vi "Main.vi"(11 "Module Admin":refnum<class "Delacor_lib_QMH_Module Admin.lvclass">) -> ()   [LabVIEW 2020, in "Acquisition.lvlib"]
doc: "This template is based off of the Queued Message Handler design pattern and the Queued Message Handler project template that ships with LabVIEW.\n\nThe main difference is that the queue is private to this module and communication between modules is performed via Broadcast and Request events.\n\nRequest events are wrapped in public API methods and are handled in the Event Handling Loop (EHL) of this VI. Any module can register for Broadcast events sent by this module. The EHL generates messages based on user interface actions.\n\nThe Message Handling Loop (MHL) processes messages generated by the EHL, or by other messages. The messages are string values, so new messages can be added easily to the Message Cases case structure in the MHL. Each message cluster can also provide an optional value for Message Data, which is a variant that can be converted to whatever message-specific data is required.\n_____\nBased on Delacor QMH Project Template 6.0.0.89."
uses:
  Acquisition.lvlib
  <vilib>/Delacor/Delacor QMH/Libraries/Module Admin_class/Delacor_lib_QMH_Module Admin.lvclass
  Shared/AnalogAcquisitionParameters__typedef.ctl
  Shared/DigitalAcquisitionParameters__typedef.ctl
  Module Data--cluster.ctl
  Stop Argument--cluster.ctl
  <vilib>/Delacor/Delacor QMH/Libraries/Message Queue_class/Delacor_lib_QMH_Message Queue.lvclass/Delacor_lib_QMH_Message Queue.ctl
  <vilib>/Delacor/Delacor QMH/Libraries/Module Admin_class/Delacor_lib_QMH_Module Admin.lvclass/Delacor_lib_QMH_Module Admin.ctl
  Start Acquisition Argument--cluster.ctl
  Configure Analog Task Acquisition Argument--cluster.ctl
  Configure Digital Taks Acquisition Argument--cluster.ctl
  Start Analog Acquisition Helper Loop Argument--cluster.ctl
  Start Digital Acquisition Helper Loop Argument--cluster.ctl
  Stop Analog Acquisition Helper Loop Argument--cluster.ctl
  Stop Digital Acquisition Helper Loop Argument--cluster.ctl
  <vilib>/DAQmx/read.llb/DAQmx Read (Digital 1D U32 NChan 1Samp).vi
  <vilib>/DAQmx/read.llb/DAQmx Read (Digital 1D Bool NChan 1Samp 1Line).vi
  <vilib>/DAQmx/read.llb/DAQmx Read (Analog 1D Wfm NChan NSamp).vi
  <vilib>/Delacor/Delacor QMH/Libraries/Message Queue_class/Delacor_lib_QMH_Enqueue Message (Single).vi
  <vilib>/Delacor/Delacor QMH/Libraries/Module Admin_class/Delacor_lib_QMH_Get External Launch.vi
  <vilib>/DAQmx/miscellaneous.llb/DAQmx Fill In Error Info.vi
  <vilib>/Utility/error.llb/Error Cluster From Error Code.vi
  <vilib>/ErrorRing/Error Ring.xnode
  <vilib>/Delacor/Delacor QMH/Libraries/Message Queue_class/Delacor_lib_QMH_Message Queue.lvclass
  Shared/Configuration for Acquisitions.lvlib
panel:
  in  "Analog - Digital":bool
  in  "Digital Acquisition Parameters":T1 {"Execution Task Frequency" scale=1.0..100.0}
  in  "Analog Acquisition Parameters":T2={"sampling frequency Analog"=1000, "number of samples Analog"=1000, "Channels Analog"=[]} {"number of samples Analog" scale=0.0..2000.0; "sampling frequency Analog" scale=0.0..2000.0}
  in  "Total Acquisition Time":i32
  in  "DAQ Device Name":tag
  out "error out":errorcluster
  in  "Start Acquisition":bool
  out "Array Datos Digitales":bool[](array[boolean])
  out "Grafica Datos Analógicos":waveform(dbl)[](graph)
  out "Status":string
  # "#LaterOn\nThis parameters are not taken from the Acquisition module, but\nreceived by it. The information comes from an external request\n(tester) or from a broadcast (Settings module)"
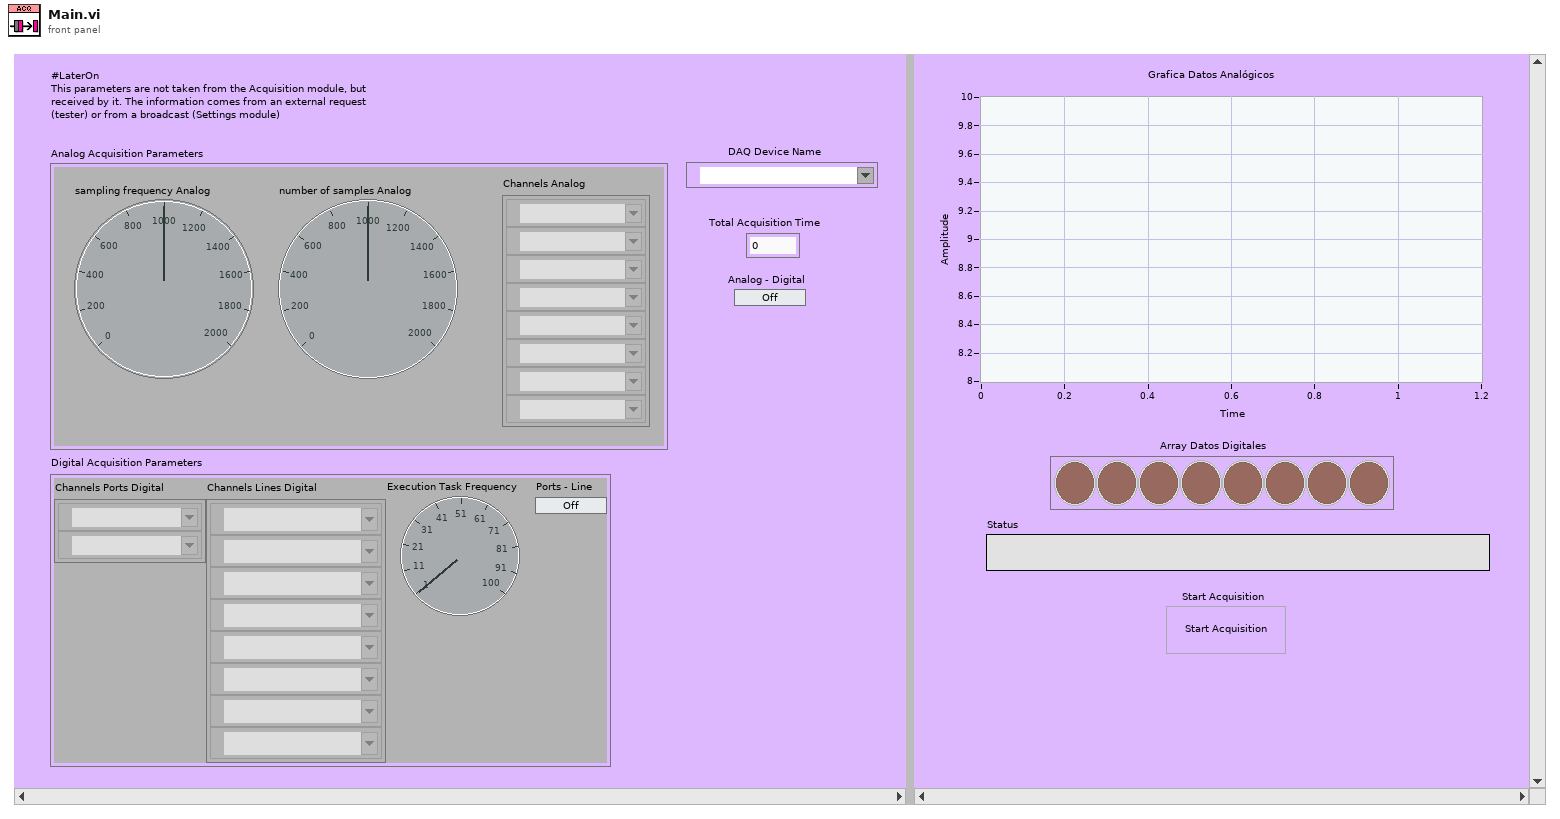
[diagram p1: front panel]
types:
  T1 = typedef "Configuration for Acquisitions.lvlib/DigitalAcquisitionParameters__typedef.ctl" = cluster{"Channels Ports Digital":tag[], "Channels Lines Digital":tag[], "Execution Task Frequency\n":u32, "Ports - Line":bool}
  T2 = typedef "Configuration for Acquisitions.lvlib/AnalogAcquisitionParameters__typedef.ctl" = cluster{"sampling frequency Analog":u32, "number of samples Analog":u32, "Channels Analog":tag[]}
  T3 = typedef "Acquisition.lvlib/Request Events--cluster.ctl" = cluster{"Stop Module":refnum<user-event>, "Show Panel":refnum<user-event>, "Hide Panel":refnum<user-event>, "Get Module Execution Status":refnum<user-event>, "Show Diagram":refnum<user-event>, "Start Acquisition":refnum<user-event>, "Configure Analog Task Acquisition":refnum<user-event>, "Configure Digital Taks Acquisition":refnum<user-event>, "Start Analog Acquisition Helper Loop":refnum<user-event>, "Start Digital Acquisition Helper Loop":refnum<user-event>, "Stop Analog Acquisition Helper Loop":refnum<user-event>, "Stop Digital Acquisition Helper Loop":refnum<user-event>}
  T4 = enum32{"invalid lock state", "Not Locked", "Locked (No Password)", "Password-protected"}
  T5 = typedef "Acquisition.lvlib/Stop Argument--cluster.ctl" = cluster{"Origin":string, "Exit via Stop Module Req?":bool, "Wait for Module to stop?":bool}
  T6 = typedef "Acquisition.lvlib/Start Acquisition Argument--cluster.ctl" = cluster{"Start Acquisition":bool, "Analog - Digital":bool}
  T7 = typedef "Acquisition.lvlib/Configure Analog Task Acquisition Argument--cluster.ctl" = cluster{"DAQ Device Name":tag, "Total Acquisition Time":i32, "Analog Acquisition Parameters":T2}
  T8 = typedef "Acquisition.lvlib/Configure Digital Taks Acquisition Argument--cluster.ctl" = cluster{"DAQ Device Name":tag, "Total Acquisition Time":i32, "Digital Acquisition Parameters":T1}
  T9 = typedef "Acquisition.lvlib/Start Analog Acquisition Helper Loop Argument--cluster.ctl" = cluster{"Analog Acq. Timeout":i32}
  T10 = typedef "Acquisition.lvlib/Start Digital Acquisition Helper Loop Argument--cluster.ctl" = cluster{"Digital Acq. Timeout":i32}
  T11 = typedef "Acquisition.lvlib/Stop Analog Acquisition Helper Loop Argument--cluster.ctl" = cluster{"Boolean":bool}
  T12 = typedef "Acquisition.lvlib/Stop Digital Acquisition Helper Loop Argument--cluster.ctl" = cluster{"Boolean":bool}
  T13 = enum32{"Invalid", "Standard", "Closed", "Hidden", "Minimized", "Maximized"}
  T14 = typedef "Acquisition.lvlib/Module Data--cluster.ctl" = cluster{"Status":string, "DAQ Device Name":tag, "Total Acquisition Time":u32, "Analog Acquisition Parameters":T2, "Digital Acquisition Parameters":T1, "Acquisition Type":bool}
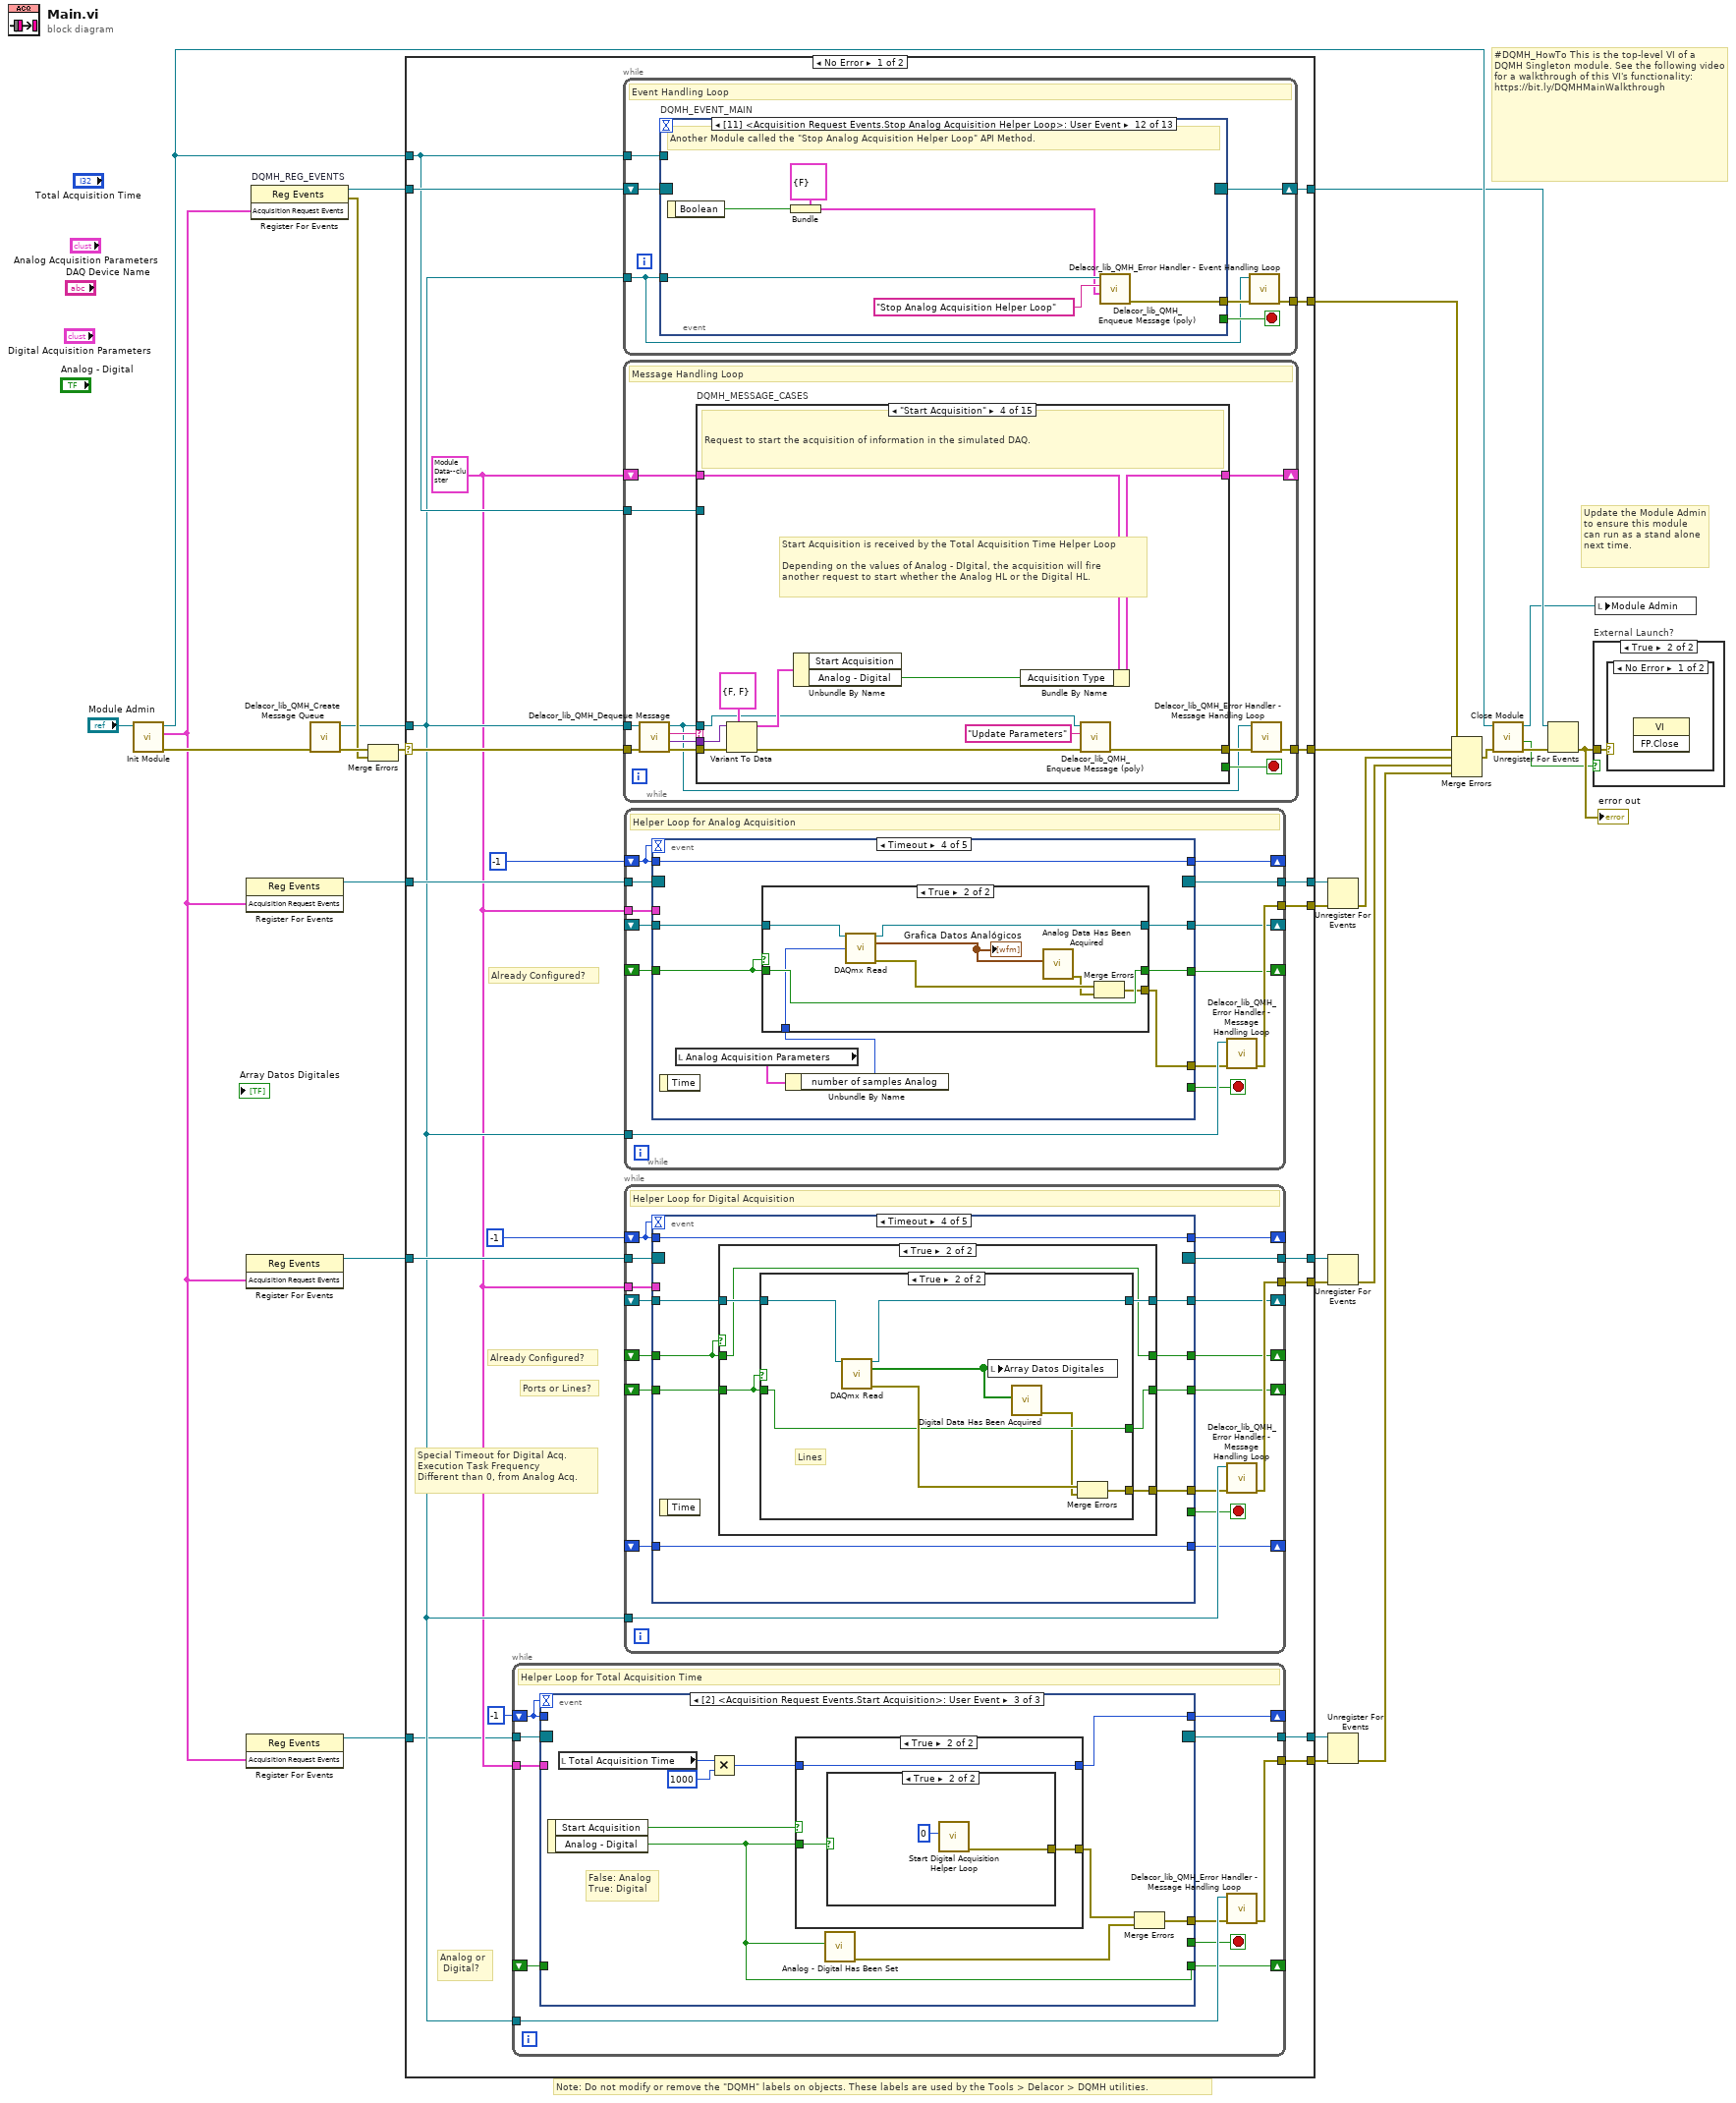
[diagram p0: block diagram]
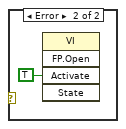
[diagram p3: hidden frame]
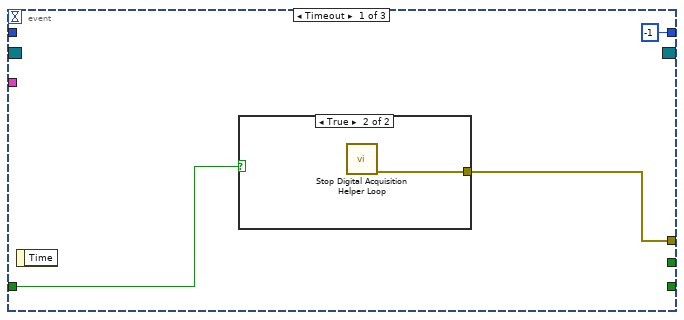
[diagram p4: hidden frame]
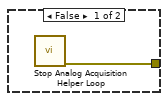
[diagram p5: hidden frame]
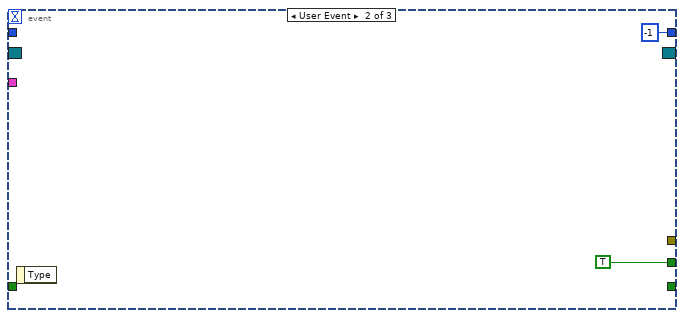
[diagram p6: hidden frame]
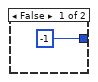
[diagram p7: hidden frame]
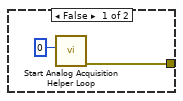
[diagram p8: hidden frame]
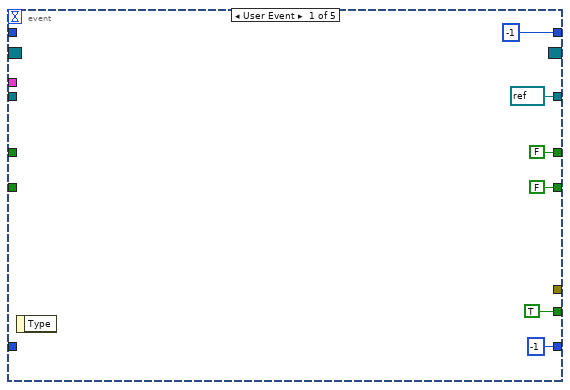
[diagram p9: hidden frame]
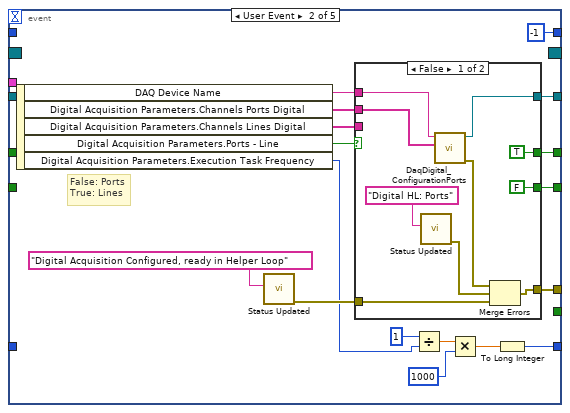
[diagram p10: hidden frame]
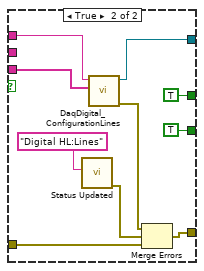
[diagram p11: hidden frame]
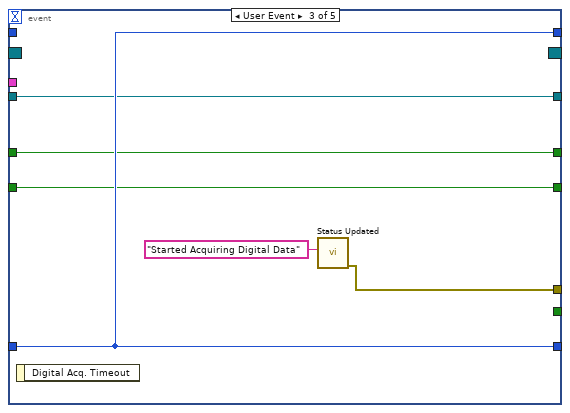
[diagram p12: hidden frame]
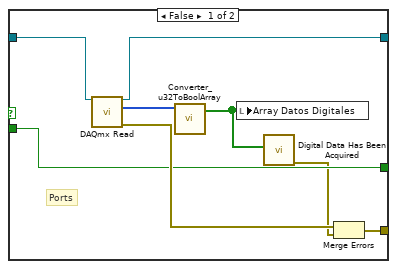
[diagram p14: hidden frame]
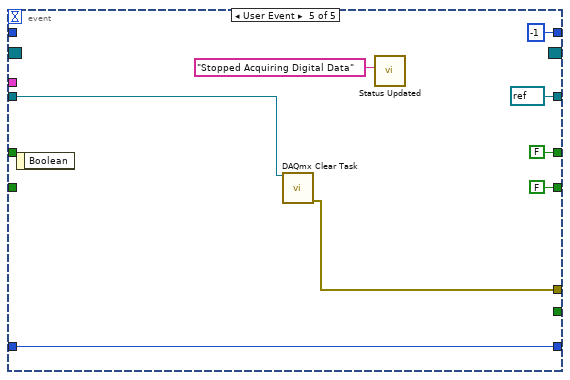
[diagram p15: hidden frame]
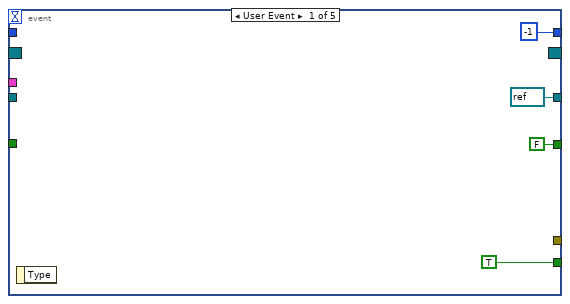
[diagram p16: hidden frame]
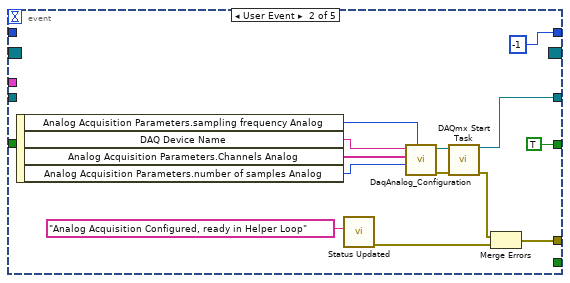
[diagram p17: hidden frame]
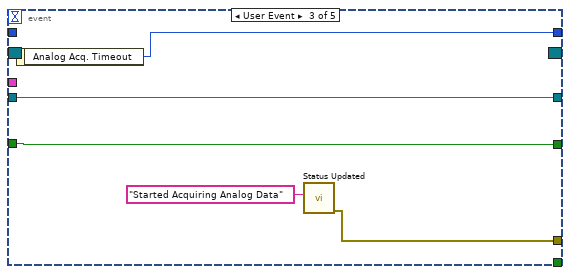
[diagram p18: hidden frame]
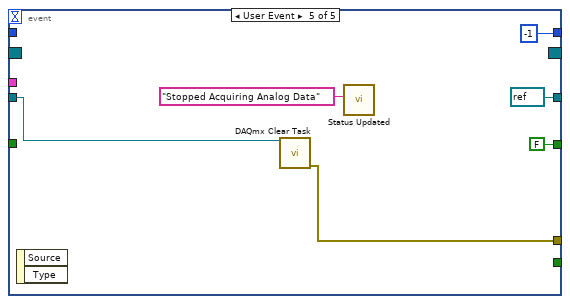
[diagram p20: hidden frame]
diagram:
  # "#DQMH_HowTo This is the top-level VI of a DQMH Singleton module. See the following video for a walkthrough of this VI's functionality: https://bit.ly/DQMHMainWalkthrough"
  # "Note: Do not modify or remove the \"DQMH\" labels on objects. These labels are used by the Tools > Delacor > DQMH utilities."
  # "Update the Module Admin to ensure this module can run as a stand alone next time."
  n1 = call "Init Module.vi"("Singleton Module Admin in"="Module Admin") -> ("error out"=w28:errorcluster, "Acquisition Request Events"=w1:T3, "Singleton Module Admin out"=w20:refnum<class "Delacor_lib_QMH_Module Admin.lvclass">)  [unwired: 8 in]
  n2 = register-events(w1) -> (reference out=w13:refnum<event-registration>)  [unwired: 2 in, 1 out]
  n3 = register-events(w1) -> (reference out=w9:refnum<event-registration>)  [unwired: 2 in, 1 out]
  n4 = register-events(w1) -> (reference out=w2:refnum<event-registration>)  [unwired: 2 in, 1 out]
  n5 = register-events "DQMH_REG_EVENTS"(w1) -> (reference out=w18:refnum<event-registration>, error out=w21:errorcluster)  [unwired: 2 in]
  n6 = call <vilib>:"Delacor_lib_QMH_Create Message Queue.vi"("error in"=w28) -> ("error out"=w23:errorcluster, "Message Queue"=w17:refnum<class "Delacor_lib_QMH_Message Queue.lvclass">)  [unwired: 9 in]
  n7 = Merge Errors(w23, w21) -> (w22:errorcluster)
  n8 = case shown="No Error" w22 {
    selector: w22 -> [w47 w507]
    tunnel: [w49 w506] -> w29
    tunnel: [w46 w512] -> w19
    tunnel: w18 -> [w45 w512]
    tunnel: w17 -> [w36 w505]
    tunnel: [w48 _] -> w26
    tunnel: w20 -> [w41 w508]
    tunnel: w13 -> [w44 w504]
    tunnel: [w43 w504] -> w12
    tunnel: [w42 _] -> w11
    tunnel: w9 -> [w40 w503]
    tunnel: [w39 w503] -> w8
    tunnel: [w38 _] -> w7
    tunnel: [w34 w502] -> w5
    tunnel: [w33 _] -> w4
    tunnel: w2 -> [w32 w502]
    frame No Error {
      w35 = T14 {"Status"="", "DAQ Device Name"="", "Total Acquisition Time"=0, "Analog Acquisition Parameters"={"sampling frequency Analog"=1000, "number of samples Analog"=1000, "Channels Analog"=[]}, "Digital Acquisition Parameters"={"Channels Ports Digital"=[], "Channels Lines Digital"=[], "Execution Task Frequency\n"=0, "Ports - Line"=FALSE}, "Acquisition Type"=FALSE} ("Data Cluster")
      # "Analog or\n Digital?"
      # "Ports or Lines?"
      # "Special Timeout for Digital Acq.\nExecution Task Frequency\nDifferent than 0, from Analog Acq."
      # "Already Configured?"
      # "Already Configured?"
      n9 = while {
        tunnel: w32 -> [w60]
        shift-right: [w58] -> _
        shift-left: -1 -> [w59]
        tunnel: w35 -> [w57]
        tunnel: [w56] -> w34
        tunnel: [w55] -> w33
        tunnel: w36 -> [w54]
        shift-right: [w51] -> _
        shift-left: _ -> [w50]
        stop <- w52 stop-if-true
        # "Helper Loop for Total Acquisition Time"
        n10 = event shown="[2] <Acquisition Request Events.Start Acquisition>: User Event" {
          selector: w60 -> [_ _ _]
          dyn-events: [_ _ _] -> w56
          timeout: w59 -> [_ _ _]
          tunnel: w59 -> [_ _ _]
          tunnel: [-1 -1 w73] -> w58
          tunnel: w57 -> [_ _ _]
          tunnel: [w62 _ w69] -> w53
          tunnel: [_ TRUE _] -> w52
          tunnel: [_ _ w70] -> w51
          tunnel: w50 -> [w63 _ _]
          event Timeout {
            n11 = event-data() -> ()  [unwired: 1 in, 1 out]
            n12 = case shown="True" w63 {
              tunnel: [w64 w65] -> w62
              frame False {
                n13 = call "Stop Analog Acquisition Helper Loop.vi"() -> ("error out"=w64:errorcluster)  [unwired: 11 in]
              }
              frame True {
                n14 = call "Stop Digital Acquisition Helper Loop.vi"() -> ("error out"=w65:errorcluster)  [unwired: 11 in]
              }
            }
          }
          event User Event {
            n15 = event-data() -> ()  [unwired: 1 in, 1 out]
          }
          event User Event {
            # "False: Analog\nTrue: Digital"
            n16 = event-data() -> ("Start Acquisition"=w76:bool, "Analog - Digital"=w70:bool)  [unwired: 1 in]
            n17 = local read "Total Acquisition Time"() -> (w74:i32)
            n18 = Multiply(x=w74, y=1000) -> (x*y=w72:i32)
            n19 = case shown="True" w76 {
              tunnel: w70 -> [_ w80]
              tunnel: [_ w79] -> w75
              tunnel: w72 -> [_ w78]
              tunnel: [-1 w78] -> w73
              frame False {
              }
              frame True {
                n20 = case shown="True" w80 {
                  tunnel: [w82 w84] -> w79
                  frame False {
                    n21 = call "Start Analog Acquisition Helper Loop.vi"("Analog Acq. Timeout"=0) -> ("error out"=w82:errorcluster)  [unwired: 10 in]
                  }
                  frame True {
                    n22 = call "Start Digital Acquisition Helper Loop.vi"("Digital Acq. Timeout"=0) -> ("error out"=w84:errorcluster)  [unwired: 10 in]
                  }
                }
              }
            }
            n23 = call "Analog - Digital Has Been Set.vi"("Analog - Digital"=w70) -> ("error out"=w68:errorcluster)  [unwired: 10 in]
            n24 = Merge Errors(w75, w68) -> (w69:errorcluster)
          }
        }
        n25 = call-dynamic "Delacor_lib_QMH_Error Handler - Message Handling Loop.vi"("error in"=w53, "Message Queue in"=w54) -> ("dup error in"=w55:errorcluster)  [unwired: 8 in, 1 out]
      }
      n26 = while {
        tunnel: w36 -> [w251]
        shift-right: [w254] -> w46
        shift-left: w45 -> [w255]
        tunnel: [w256] -> w48
        tunnel: w41 -> [w252]
        stop <- w253 stop-if-true
        # "Event Handling Loop"
        n27 = event "DQMH_EVENT_MAIN" shown="[11] <Acquisition Request Events.Stop Analog Acquisition Helper Loop>: User Event" {
          selector: w255 -> [_ _ _ _ _ _ _ _ _ _ _ _ _]
          dyn-events: [_ _ _ _ _ _ _ _ _ _ _ _ _] -> w254
          timeout: _ -> [_ _ _ _ _ _ _ _ _ _ _ _ _]
          tunnel: [_ _ _ _ TRUE ("Discard?") _ _ _ _ _ _ _ _] -> w253
          tunnel: w251 -> [_ _ _ _ w280 w287 w301 w309 w317 w323 w329 w335 w341]
          tunnel: [_ _ w263 _ w283 w289 w296 w302 w310 w318 w324 w330 w336] -> w257
          tunnel: w252 -> [_ _ _ _ _ w286 _ _ _ _ _ _ _]
          event User Event {
            # "Show the panel of this VI, and send a status updated message to let listeners know."
            # "Another Module called the \"Show Panel\" API Method."
            n28 = event-data() -> ()  [unwired: 1 in, 1 out]
            n29 = control-ref of="This VI"() -> (w259:refnum<vi>)
            n30 = call "Open VI Panel.vi"("VI"=w259) -> ()  [unwired: 10 in, 1 out]
            n31 = call "Status Updated.vi"("Status"="Panel shown." ("format string")) -> ()  [unwired: 10 in, 1 out]
          }
          event User Event {
            # "Hide the panel of this VI, and send a status updated message to let listeners know."
            # "Another Module called the \"Hide Panel\" API Method."
            n32 = event-data() -> ()  [unwired: 1 in, 1 out]
            n33 = control-ref of="This VI"() -> (w261:refnum<vi>)
            n34 = call "Hide VI Panel.vi"("VI"=w261) -> ()  [unwired: 10 in, 1 out]
            n35 = call "Status Updated.vi"("Status"="Panel hidden." ("format string")) -> ()  [unwired: 10 in, 1 out]
          }
          event User Event {
            # "Another Module called the \"Get Module Execution Status\" API Method."
            n36 = event-data() -> ()  [unwired: 1 in, 1 out]
            n37 = call "Update Module Execution Status.vi"("Running?"=TRUE) -> ("error out"=w263:errorcluster)  [unwired: 10 in]
          }
          event User Event {
            # "Another Module called the \"Show Diagram\" API Method. This event is used for debugging."
            n38 = event-data() -> ()  [unwired: 1 in, 1 out]
            n39 = disable-structure shown="RUN_TIME_ENGINE==False" {
              frame condition #0 (active) {
                # "functionality not available in exe"
                n40 = invoke class="VI" method="Lock State.Get"() -> (error out=w269:errorcluster, "Get Lock State"=w268:T4, "pwd in cache"=w265:bool)  [unwired: 4 in, 1 out]
                n41 = Equal?(x=T4."Password-protected", y=w268) -> (x = y?=w266:bool)
                n42 = Compound Arithmetic op=AND(w266, invert w265) -> (w264:bool)
                n43 = case shown="False" w264 {
                  tunnel: w269 -> [w272 _]
                  frame False {
                    n44 = property class="VI"(error in=w272, "BDWin.Open"=TRUE ("Block Diagram Window:Open")) -> ()  [unwired: 1 in, 2 out]
                    n45 = call "Status Updated.vi"("Status"="Block Diagram shown." ("format string")) -> ()  [unwired: 10 in, 1 out]
                  }
                  frame True {
                    # "Password-protected VI, and the password is not in the cache. Do not show the diagram."
                  }
                }
              }
              frame condition #1 {
              }
            }
          }
          event User Event {
            # "The Stop Module Event can get fired from the Exit message in the MHL. The queue gets destroyed in that case. If the queue no longer exists, the Enqueue Exit as a priority message will return error 1. It is safe to ignore, because the module is already exiting."
            # "Another Module called the \"Stop Module\" API Method  or the Message Handling Loop below."
            n46 = event-data() -> ("Origin"=w279:string, "Exit via Stop Module Req?"=w275:bool, "Wait for Module to stop?"=w274:bool)  [unwired: 1 in]
            n47 = local write "Status"(w279) -> ()
            n48 = Bundle By Name(cluster=T5 {"Origin"="", "Exit via Stop Module Req?"=FALSE, "Wait for Module to stop?"=FALSE} ("Stop Argument"), "Exit via Stop Module Req?"=w275, "Wait for Module to stop?"=w274) -> (w273:T5)
            n49 = call-poly <vilib>:"Delacor_lib_QMH_Enqueue Message (poly).vi"("Priority Message? (F)"=TRUE, "Message Data"=w273, "Message"="Exit", "Message Queue in"=w280) -> ("error out"=w284:errorcluster)  [unwired: 6 in, 1 out]
            n50 = call <vilib>:"Clear Errors.vi"("error in (no error)"=w284, "specific error code to clear (0: all)"=1) -> ("error out"=w283:errorcluster)  [unwired: 4 in, 1 out]
          }
          event Panel Close? {
            w288 = TRUE  # Discard the event, the MHL is responsible for closing and stopping this VI.
            # "Hide the panel or send the 'Exit' message if the user clicks the 'X' on the module main VI panel."
            n51 = event-data() -> ()  [unwired: 1 in, 1 out]
            n52 = property class="Module Admin"(reference=w286) -> ("Accessors:External Launch"=w285:bool)  [unwired: 1 in, 2 out]
            n53 = case shown="False" w285 {
              tunnel: w287 -> [_ w293]
              tunnel: [_ w294] -> w289
              frame True {
                # "If externally launched, clicking the 'X' hides the panel, but doesn't close it."
                n54 = control-ref of="This VI"() -> (w290:refnum<vi>)
                n55 = call "Hide VI Panel.vi"("VI"=w290) -> ()  [unwired: 10 in, 1 out]
              }
              frame False {
                # "If run as a stand-alone VI, clicking the panel 'X' stops the VI."
                n56 = call-poly <vilib>:"Delacor_lib_QMH_Enqueue Message (poly).vi"("Priority Message? (F)"=TRUE, "Message"="Exit", "Message Queue in"=w293) -> ("error out"=w294:errorcluster)  [unwired: 7 in, 1 out]
              }
            }
            n57 = event-data("Discard?"=w288) -> ()  [unwired: 1 in, 1 out]
          }
          event User Event {
            # "Another Module called the \"Start Acquisition\" API Method."
            n58 = event-data() -> ("Start Acquisition"=w297:bool, "Analog - Digital"=w295:bool)  [unwired: 1 in]
            n59 = Bundle(cluster=T6 {"Start Acquisition"=FALSE, "Analog - Digital"=FALSE} ("Start Acquisition Argument"), "Start Acquisition"=w297, "Analog - Digital"=w295) -> (w298:T6)
            n60 = call-poly <vilib>:"Delacor_lib_QMH_Enqueue Message (poly).vi"("Message Data"=w298, "Message"="Start Acquisition", "Message Queue in"=w301) -> ("error out"=w296:errorcluster)  [unwired: 7 in, 1 out]
          }
          event User Event {
            # "Another Module called the \"Configure Analog Task Acquisition\" API Method."
            n61 = event-data() -> ("DAQ Device Name"=w305:tag, "Total Acquisition Time"=w304:i32, "Analog Acquisition Parameters"=w303:T2)  [unwired: 1 in]
            n62 = Bundle(cluster=T7 {"DAQ Device Name"="", "Total Acquisition Time"=0, "Analog Acquisition Parameters"={"sampling frequency Analog"=1000, "number of samples Analog"=1000, "Channels Analog"=[]}} ("Configure Analog Task Acquisition Argument"), "DAQ Device Name"=w305, "Total Acquisition Time"=w304, "Analog Acquisition Parameters"=w303) -> (w306:T7)
            n63 = call-poly <vilib>:"Delacor_lib_QMH_Enqueue Message (poly).vi"("Message Data"=w306, "Message"="Configure Analog Task Acquisition", "Message Queue in"=w309) -> ("error out"=w302:errorcluster)  [unwired: 7 in, 1 out]
          }
          event User Event {
            # "Another Module called the \"Configure Digital Taks Acquisition\" API Method."
            n64 = event-data() -> ("DAQ Device Name"=w313:tag, "Total Acquisition Time"=w312:i32, "Digital Acquisition Parameters"=w311:T1)  [unwired: 1 in]
            n65 = Bundle(cluster=T8 {"DAQ Device Name"="", "Total Acquisition Time"=0, "Digital Acquisition Parameters"={"Channels Ports Digital"=[], "Channels Lines Digital"=[], "Execution Task Frequency\n"=0, "Ports - Line"=FALSE}} ("Configure Digital Taks Acquisition Argument"), "DAQ Device Name"=w313, "Total Acquisition Time"=w312, "Digital Acquisition Parameters"=w311) -> (w314:T8)
            n66 = call-poly <vilib>:"Delacor_lib_QMH_Enqueue Message (poly).vi"("Message Data"=w314, "Message"="Configure Digital Taks Acquisition", "Message Queue in"=w317) -> ("error out"=w310:errorcluster)  [unwired: 7 in, 1 out]
          }
          event User Event {
            # "Another Module called the \"Start Analog Acquisition Helper Loop\" API Method."
            n67 = event-data() -> ("Analog Acq. Timeout"=w319:i32)  [unwired: 1 in]
            n68 = Bundle(cluster=T9 {"Analog Acq. Timeout"=0} ("Start Analog Acquisition Helper Loop Argument"), "Analog Acq. Timeout"=w319) -> (w320:T9)
            n69 = call-poly <vilib>:"Delacor_lib_QMH_Enqueue Message (poly).vi"("Message Data"=w320, "Message"="Start Analog Acquisition Helper Loop", "Message Queue in"=w323) -> ("error out"=w318:errorcluster)  [unwired: 7 in, 1 out]
          }
          event User Event {
            # "Another Module called the \"Start Digital Acquisition Helper Loop\" API Method."
            n70 = event-data() -> ("Digital Acq. Timeout"=w325:i32)  [unwired: 1 in]
            n71 = Bundle(cluster=T10 {"Digital Acq. Timeout"=0} ("Start Digital Acquisition Helper Loop Argument"), "Digital Acq. Timeout"=w325) -> (w326:T10)
            n72 = call-poly <vilib>:"Delacor_lib_QMH_Enqueue Message (poly).vi"("Message Data"=w326, "Message"="Start Digital Acquisition Helper Loop", "Message Queue in"=w329) -> ("error out"=w324:errorcluster)  [unwired: 7 in, 1 out]
          }
          event User Event {
            # "Another Module called the \"Stop Analog Acquisition Helper Loop\" API Method."
            n73 = event-data() -> ("Boolean"=w331:bool)  [unwired: 1 in]
            n74 = Bundle(cluster=T11 {"Boolean"=FALSE} ("Stop Analog Acquisition Helper Loop Argument"), "Boolean"=w331) -> (w332:T11)
            n75 = call-poly <vilib>:"Delacor_lib_QMH_Enqueue Message (poly).vi"("Message Data"=w332, "Message"="Stop Analog Acquisition Helper Loop", "Message Queue in"=w335) -> ("error out"=w330:errorcluster)  [unwired: 7 in, 1 out]
          }
          event User Event {
            # "Another Module called the \"Stop Digital Acquisition Helper Loop\" API Method."
            n76 = event-data() -> ("Boolean"=w337:bool)  [unwired: 1 in]
            n77 = Bundle(cluster=T12 {"Boolean"=FALSE} ("Stop Digital Acquisition Helper Loop Argument"), "Boolean"=w337) -> (w338:T12)
            n78 = call-poly <vilib>:"Delacor_lib_QMH_Enqueue Message (poly).vi"("Message Data"=w338, "Message"="Stop Digital Acquisition Helper Loop", "Message Queue in"=w341) -> ("error out"=w336:errorcluster)  [unwired: 7 in, 1 out]
          }
        }
        n79 = call-dynamic "Delacor_lib_QMH_Error Handler - Event Handling Loop.vi"("error in"=w257, "Message Queue in"=w251) -> ("dup error in"=w256:errorcluster)  [unwired: 8 in, 1 out]
      }
      n80 = while {
        tunnel: w36 -> [w344]
        shift-right: [w348] -> _
        shift-left: w35 -> [w349]
        tunnel: w47 -> [w352]
        tunnel: [w350] -> w49
        tunnel: w41 -> [w342]
        stop <- w347 stop-if-true
        # "Message Handling Loop"
        n81 = call-dynamic "Delacor_lib_QMH_Dequeue Message.vi"("error in"=w352, "Message Queue in"=w344) -> ("error out"=w351:errorcluster, "Message Data"=w345:variant, "Message"=w346:string, "Message Queue out"=w343:refnum<class "Delacor_lib_QMH_Message Queue.lvclass">)  [unwired: 6 in]
        n82 = case "DQMH_MESSAGE_CASES" shown="\"Start Acquisition\"" w346 {
          selector: w346 -> [_ _ _ _ _ _ _ _ _ _ _ _ _ _ w489]
          tunnel: w343 -> [_ _ _ w385 w399 w416 _ _ _ _ _ _ w459 w481 _]
          tunnel: w351 -> [w370 w376 w384 w395 w411 w427 w433 w439 w445 w451 w454 w456 w466 w487 w491]
          tunnel: [w368 w376 w384 w387 w397 w413 w431 w437 w443 w449 w453 w456 w462 w484 w492] -> w353
          tunnel: w349 -> [w359 w375 w383 w391 w407 w423 w432 w438 w444 w450 w452 w455 w461 w480 w490]
          tunnel: [w358 w375 w383 w389 w406 w419 w432 w438 w444 w450 w452 w455 w461 w480 w490] -> w348
          tunnel: [_ _ _ _ _ _ _ _ _ _ _ _ _ w479 _] -> w347
          tunnel: w345 -> [_ _ _ w394 w410 w426 w430 w436 w442 w448 _ _ w460 w478 _]
          tunnel: w342 -> [w360 _ _ _ _ _ _ _ _ _ _ _ w458 w473 _]
          frame "Initialize" {
            w354 = "Initial Message" ("Initial Message")
            # "#CodeNeeded - Initialize the appearance of the front panel."
            # "#CodeNeeded - Initialize your state data here."
            # "Initialize - Any operation that needs to be done before the module can receive messages. Synchronize Caller Events.vi will inform Start Module.vi that the module has launched and is ready to receive messages. Module Did Init.vi will broadcast that the module initialized."
            n83 = call "Synchronize Caller Events.vi"("error in (no error)"=w370, "Singleton Module Admin in"=w360) -> ("error out"=w369:errorcluster, "Singleton Module Admin out"=w355:refnum<class "Delacor_lib_QMH_Module Admin.lvclass">)  [unwired: 8 in]
            n84 = property class="Module Admin"(reference=w355) -> ("Accessors:External Launch"=w364:bool)  [unwired: 1 in, 2 out]
            n85 = Select(t=T13."Hidden" ("State"), s=w364, f=T13."Standard" ("State")) -> (s? t:f=w361:T13)
            n86 = call "Module Name--constant.vi"() -> ("Module Name"=w367:string)  [unwired: 11 in]
            n87 = property class="VI"("Front Panel.Title"=w367) -> (reference out=w366:refnum<vi>, error out=w372:errorcluster)  [unwired: 2 in]
            n88 = call "Module Name--constant.vi"() -> ("Module Name"=w356:string)  [unwired: 11 in]
            n89 = invoke class="VI" method="FP.Open"(reference=w366, error in=w372, "State"=w361) -> (reference out=w365:refnum<vi>, error out=w371:errorcluster)  [unwired: 2 in, 3 out]
            n90 = Bundle By Name(cluster=w359, "Status"=w354) -> (w358:T14)
            n91 = call "Module Did Init.vi"("error in (no error)"=w369, "Initialized?"=TRUE, "Origin"=w356) -> ("error out"=w368:errorcluster)  [unwired: 8 in]
            n92 = invoke class="VI" method="FP.Center"(reference=w365, error in=w371) -> ()  [unwired: 1 in, 3 out]
            "Status" <- w354
          }
          frame "---Module Specific---" {
            # "Separator -- The following cases handle messages specific to this Module."
            n93 = Unbundle By Name(w375) -> ("Analog Acquisition Parameters"=w373:T2, "Digital Acquisition Parameters"=w374:T1)  [unwired: 3 out]
            n94 = Unbundle By Name(w374) -> ()  [unwired: 4 out]
            n95 = Unbundle By Name(w373) -> ()  [unwired: 3 out]
          }
          frame "Update Parameters" {
            n96 = Unbundle By Name(w383) -> ("Status"=w382:string, "DAQ Device Name"=w381:tag, "Total Acquisition Time"=w380:u32, "Analog Acquisition Parameters"=w378:T2, "Digital Acquisition Parameters"=w379:T1, "Acquisition Type"=w377:bool)
            n97 = local write "Status"(w382) -> ()
            n98 = local write "DAQ Device Name"(w381) -> ()
            n99 = local write "Total Acquisition Time"(w380) -> ()
            n100 = local write "Analog Acquisition Parameters"(w378) -> ()
            n101 = local write "Digital Acquisition Parameters"(w379) -> ()
            n102 = local write "Analog - Digital"(w377) -> ()
          }
          frame "Start Acquisition" {
            # "Start Acquisition is received by the Total Acquisition Time Helper Loop\n\nDepending on the values of Analog - DIgital, the acquisition will fire\nanother request to start whether the Analog HL or the Digital HL."
            # "Request to start the acquisition of information in the simulated DAQ."
            n103 = Variant To Data(error in=w395, type=T6 {"Start Acquisition"=FALSE, "Analog - Digital"=FALSE} ("Start Acquisition Argument"), Variant=w394) -> (data=w392:T6, error out=w386:errorcluster)
            n104 = Unbundle By Name(w392) -> ("Analog - Digital"=w390:bool)  [unwired: 1 out]
            n105 = Bundle By Name(cluster=w391, "Acquisition Type"=w390) -> (w389:T14)
            n106 = call-poly <vilib>:"Delacor_lib_QMH_Enqueue Message (poly).vi"("error in"=w386, "Message"="Update Parameters", "Message Queue in"=w385) -> ("error out"=w387:errorcluster)  [unwired: 7 in, 1 out]
          }
          frame "Configure Analog Task Acquisition" {
            w398 = "Analog Task Configured" ("Status")
            # "The Information has been passed to the request parameters. The Helper Loop will \ntake the information pushed through the request module to Configure the DAQ\nat the Helper Loop for acquisition."
            # "Request to configure all the parameters needed for the Analog Acquisition to be realized by its Helper Loop."
            n107 = Variant To Data(error in=w411, type=T7 {"DAQ Device Name"="", "Total Acquisition Time"=0, "Analog Acquisition Parameters"={"sampling frequency Analog"=1000, "number of samples Analog"=1000, "Channels Analog"=[]}} ("Configure Analog Task Acquisition Argument"), Variant=w410) -> (data=w408:T7, error out=w400:errorcluster)
            n108 = Unbundle By Name(w408) -> ("DAQ Device Name"=w405:tag, "Total Acquisition Time"=w404:i32, "Analog Acquisition Parameters"=w403:T2)
            n109 = Bundle By Name(cluster=w407, "DAQ Device Name"=w405, "Total Acquisition Time"=w404, "Analog Acquisition Parameters"=w403, "Status"=w398) -> (w406:T14)
            n110 = call "Status Updated.vi"("Status"=w398) -> ("error out"=w396:errorcluster)  [unwired: 10 in]
            n111 = call-poly <vilib>:"Delacor_lib_QMH_Enqueue Message (poly).vi"("error in"=w400, "Message"="Update Parameters", "Message Queue in"=w399) -> ("error out"=w401:errorcluster)  [unwired: 7 in, 1 out]
            n112 = Merge Errors(w401, w396) -> (w397:errorcluster)
          }
          frame "Configure Digital Taks Acquisition" {
            w414 = "Digital Task Configured" ("Status")
            # "The Information has been passed to the request parameters. The Helper Loop will \ntake the information pushed through the request module to Configure the DAQ\nat the Helper Loop for acquisition."
            # "Request to configure all the parameters needed for the Analog Acquisition to be realized by its Helper Loop."
            n113 = Variant To Data(error in=w427, type=T8 {"DAQ Device Name"="", "Total Acquisition Time"=0, "Digital Acquisition Parameters"={"Channels Ports Digital"=[], "Channels Lines Digital"=[], "Execution Task Frequency\n"=0, "Ports - Line"=FALSE}} ("Configure Digital Taks Acquisition Argument"), Variant=w426) -> (data=w424:T8, error out=w417:errorcluster)
            n114 = Unbundle By Name(w424) -> ("DAQ Device Name"=w422:tag, "Total Acquisition Time"=w421:i32, "Digital Acquisition Parameters"=w420:T1)
            n115 = Bundle By Name(cluster=w423, "DAQ Device Name"=w422, "Total Acquisition Time"=w421, "Digital Acquisition Parameters"=w420, "Status"=w414) -> (w419:T14)
            n116 = call "Status Updated.vi"("Status"=w414) -> ("error out"=w412:errorcluster)  [unwired: 10 in]
            n117 = call-poly <vilib>:"Delacor_lib_QMH_Enqueue Message (poly).vi"("error in"=w417, "Message"="Update Parameters", "Message Queue in"=w416) -> ("error out"=w418:errorcluster)  [unwired: 7 in, 1 out]
            n118 = Merge Errors(w418, w412) -> (w413:errorcluster)
          }
          frame "Start Analog Acquisition Helper Loop" {
            # "This request is private. This case and the event should be erased\nas only one module (the Total Acquisition Helper Loop), should handle it."
            # "Private request to start the Helper Loop of the Analog Acquisition task-manager."
            n119 = Variant To Data(error in=w433, type=T9 {"Analog Acq. Timeout"=0} ("Start Analog Acquisition Helper Loop Argument"), Variant=w430) -> (data=w428:T9, error out=w431:errorcluster)
            n120 = Unbundle By Name(w428) -> ()  [unwired: 1 out]
          }
          frame "Start Digital Acquisition Helper Loop" {
            # "This request is private. This case and the event should be erased\nas only one module (the Total Acquisition Helper Loop), should handle it."
            # "Private request to start the Helper Loop of the Digital Acquisition task-manager."
            n121 = Variant To Data(error in=w439, type=T10 {"Digital Acq. Timeout"=0} ("Start Digital Acquisition Helper Loop Argument"), Variant=w436) -> (data=w434:T10, error out=w437:errorcluster)
            n122 = Unbundle By Name(w434) -> ()  [unwired: 1 out]
          }
          frame "Stop Analog Acquisition Helper Loop" {
            # "This request is private. This case and the event should be erased\nas only one module (the Total Acquisition Helper Loop), should handle it."
            # "Private request to stop the Helper Loop of the Analog Acquisition task-manager."
            n123 = Variant To Data(error in=w445, type=T11 {"Boolean"=FALSE} ("Stop Analog Acquisition Helper Loop Argument"), Variant=w442) -> (data=w440:T11, error out=w443:errorcluster)
            n124 = Unbundle By Name(w440) -> ()  [unwired: 1 out]
          }
          frame "Stop Digital Acquisition Helper Loop" {
            # "This request is private. This case and the event should be erased\nas only one module (the Total Acquisition Helper Loop), should handle it."
            # "Private request to stop the Helper Loop of the Analog Acquisition task-manager."
            n125 = Variant To Data(error in=w451, type=T12 {"Boolean"=FALSE} ("Stop Digital Acquisition Helper Loop Argument"), Variant=w448) -> (data=w446:T12, error out=w449:errorcluster)
            n126 = Unbundle By Name(w446) -> ()  [unwired: 1 out]
          }
          frame "---Copy This Frame---" {
            # "Duplicate this frame when creating new messages.  Change this comment in the duplicated frame to describe this message."
            n127 = Merge Errors(w454) -> (w453:errorcluster)
          }
          frame "---Exit and Error Handling---" {
            # "Separator - The following cases handle errors and exit messages."
          }
          frame "Error" {
            # "#CodeRecommended - If you ever change the name of this \"Error\" message, you'll need to update the name in the Check Loop Error.vi as well."
            # "#CodeRecommended - If the module is running in standalone mode (External Launch = FALSE), this code will pop up an error dialog and call the 'Exit' message if an error occurs. Add more fine-grained error handling here."
            # "Error - Check the error message data and respond accordingly. This message is sent by the \"Error Handler\" VIs at the end of each loop in this application."
            n128 = property class="Module Admin"(reference=w458) -> ("Accessors:External Launch"=w457:bool)  [unwired: 1 in, 2 out]
            n129 = Variant To Data(error in=w466, type=errorcluster {"status"=FALSE, "code"=0, "source"=""} ("error constant"), Variant=w460) -> (data=w467:errorcluster, error out=w464:errorcluster)
            n130 = call "Error Reported.vi"("Error"=w467) -> ()  [unwired: 10 in, 1 out]
            n131 = case shown="False" w457 {
              tunnel: [w472 _] -> w463
              tunnel: w459 -> [w470 _]
              tunnel: w467 -> [w471 _]
              frame False {
                # "If the module is running standalone, then pop up an error dialog and call the \"Exit\" message."
                n132 = call <vilib>:"Simple Error Handler.vi"("error in (no error)"=w471) -> ()  [unwired: 4 in, 5 out]
                n133 = call-poly <vilib>:"Delacor_lib_QMH_Enqueue Message (poly).vi"("Priority Message? (F)"=TRUE, "Message"="Exit", "Message Queue in"=w470) -> ("error out"=w472:errorcluster)  [unwired: 7 in, 1 out]
              }
              frame True {
                # "If the module was launched externally, calling the Error Reported broadcast VI is the only action performed by the \"Error\" message. The module's caller can then process the error appropriately."
              }
            }
            n134 = Merge Errors(w464, w463) -> (w462:errorcluster)
            n135 = local write "error out"(w462) -> ()
          }
          frame "Exit" {
            w477 = 91  # 91: not all Exit messages will have an argument
            w479 = TRUE  # Stop the VI
            # "Release the message queue reference"
            # "#CodeNeeded - Add any required cleanup code here"
            # "Exit - Exit the application."
            n136 = Variant To Data(error in=w487, type=T5 {"Origin"="", "Exit via Stop Module Req?"=FALSE, "Wait for Module to stop?"=FALSE} ("Stop Argument"), Variant=w478) -> (data=w475:T5, error out=w483:errorcluster)
            n137 = call <vilib>:"Clear Errors.vi"("error in (no error)"=w483, "specific error code to clear (0: all)"=w477) -> ("error out"=w486:errorcluster)  [unwired: 4 in, 1 out]
            n138 = control-ref of="This VI"() -> (w474:refnum<vi>)
            n139 = call-dynamic "Delacor_lib_QMH_Release Message Queue.vi"("error in"=w486, "Message Queue"=w481) -> ("error out"=w485:errorcluster)  [unwired: 9 in]
            n140 = call "Handle Exit.vi"("Stop Argument"=w475, "Admin in"=w473, "VI reference"=w474) -> ("error out"=w482:errorcluster)  [unwired: 7 in, 1 out]
            n141 = Merge Errors(w485, w482) -> (w484:errorcluster)
          }
          frame Default {
            # "'Default' case only runs if there is a message that isn't defined in any of the other cases.  Output a programming error."
            n142 = call "Module Name--constant.vi"() -> ("Module Name"=w488:string)  [unwired: 11 in]
            n143 = xnode "Error Ring"("parameter 0"=w489, "parameter 1"=w488) -> ("error out"=w493:errorcluster)
            n144 = Merge Errors(w491, w493) -> (w492:errorcluster)
          }
        }
        n145 = call-dynamic "Delacor_lib_QMH_Error Handler - Message Handling Loop.vi"("error in"=w353, "Message Queue in"=w343) -> ("dup error in"=w350:errorcluster)  [unwired: 8 in, 1 out]
      }
      n146 = while {
        tunnel: w44 -> [w204]
        shift-right: [w202] -> _
        shift-left: -1 -> [w203]
        tunnel: w35 -> [w201]
        tunnel: [w200] -> w43
        tunnel: [w199] -> w42
        tunnel: w36 -> [w198]
        shift-right: [w195] -> _
        shift-left: _ -> [w192]
        shift-right: [w194] -> _
        shift-left: _ -> [w193]
        stop <- w196 stop-if-true
        # "Helper Loop for Analog Acquisition"
        n147 = event shown="[3] Timeout" {
          selector: w204 -> [_ _ _ _ _]
          dyn-events: [_ _ _ _ _] -> w200
          timeout: w203 -> [_ _ _ _ _]
          tunnel: w203 -> [_ _ _ w234 _]
          tunnel: [-1 -1 w224 w234 -1] -> w202
          tunnel: w201 -> [_ _ _ _ _]
          tunnel: [_ w214 w222 w227 w249] -> w197
          tunnel: [TRUE _ _ _ _] -> w196
          tunnel: [refnum<k21> refnum ("task out") w210 w226 w232 refnum<k21> refnum ("task out")] -> w195
          tunnel: [FALSE TRUE w225 w230 FALSE] -> w194
          tunnel: w193 -> [_ _ w225 w231 _]
          tunnel: w192 -> [_ _ w226 w233 w250]
          event User Event {
            n148 = event-data() -> ()  [unwired: 1 in, 1 out]
          }
          event User Event {
            n149 = event-data() -> ("Analog Acquisition Parameters.sampling frequency Analog"=w221:u32, "DAQ Device Name"=w220:tag, "Analog Acquisition Parameters.Channels Analog"=w219:tag[], "Analog Acquisition Parameters.number of samples Analog"=w218:u32)  [unwired: 1 in]
            n150 = call "Status Updated.vi"("Status"="Analog Acquisition Configured, ready in Helper Loop") -> ("error out"=w213:errorcluster)  [unwired: 10 in]
            n151 = call "DaqAnalog_Configuration.vi"("Sampling Frequency"=w221, "Number of Samples"=w218, "Canales"=w219, "DAQ Board Name"=w220) -> ("error out"=w212:errorcluster, "task out"=w211:refnum<k21>)  [unwired: 6 in]
            n152 = call <vilib>:"DAQmx Start Task.vi"("task/channels in"=w211, "error in"=w212) -> ("task out"=w210:refnum<k21>, "error out"=w209:errorcluster)  [unwired: 12 in]
            n153 = Merge Errors(w209, w213) -> (w214:errorcluster)
          }
          event User Event {
            n154 = event-data() -> ("Analog Acq. Timeout"=w224:i32)  [unwired: 1 in]
            n155 = call "Status Updated.vi"("Status"="Started Acquiring Analog Data") -> ("error out"=w222:errorcluster)  [unwired: 10 in]
          }
          event Timeout {
            n156 = event-data() -> ()  [unwired: 1 in, 1 out]
            n157 = local read "Analog Acquisition Parameters"() -> (w229:T2)
            n158 = Unbundle By Name(w229) -> ("number of samples Analog"=w228:u32)
            n159 = case shown="True" w231 {
              tunnel: w233 -> [w236 w244]
              tunnel: [w236 w243] -> w232
              tunnel: w231 -> [w235 w242]
              tunnel: [w235 w242] -> w230
              tunnel: w228 -> [_ w241]
              tunnel: [_ w238] -> w227
              frame False {
                # "This case determines whether the task has been configured, thus\nallows the system to start acquisition or ignores it."
              }
              frame True {
                n160 = call-poly <vilib>:"DAQmx Read.vi"("task/channels in"=w244, "number of samples per channel"=w241) -> ("task out"=w243:refnum<k21>, "data"=w239:waveform(dbl)[], "error out"=w240:errorcluster)  [unwired: 11 in]
                "Grafica Datos Analógicos" <- w239
                n161 = call "Analog Data Has Been Acquired.vi"("Analog Data Acq."=w239) -> ("error out"=w237:errorcluster)  [unwired: 10 in]
                n162 = Merge Errors(w240, w237) -> (w238:errorcluster)
              }
            }
          }
          event User Event {
            n163 = event-data() -> ()  [unwired: 1 in, 2 out]
            n164 = call <vilib>:"DAQmx Clear Task.vi"("task in"=w250) -> ("error out"=w249:errorcluster)  [unwired: 14 in]
            n165 = call "Status Updated.vi"("Status"="Stopped Acquiring Analog Data") -> ()  [unwired: 10 in, 1 out]
          }
        }
        n166 = call-dynamic "Delacor_lib_QMH_Error Handler - Message Handling Loop.vi"("error in"=w197, "Message Queue in"=w198) -> ("dup error in"=w199:errorcluster)  [unwired: 8 in, 1 out]
      }
      n167 = while {
        tunnel: w40 -> [w101]
        shift-right: [w99] -> _
        shift-left: -1 -> [w100]
        tunnel: w35 -> [w98]
        tunnel: [w97] -> w39
        tunnel: [w96] -> w38
        tunnel: w36 -> [w95]
        shift-right: [w92] -> _
        shift-left: _ -> [w89]
        shift-right: [w91] -> _
        shift-left: _ -> [w90]
        shift-right: [w85] -> _
        shift-left: _ -> [w88]
        shift-right: [w87] -> _
        shift-left: _ -> [w86]
        stop <- w93 stop-if-true
        # "Helper Loop for Digital Acquisition"
        n168 = event shown="[3] Timeout" {
          selector: w101 -> [_ _ _ _ _]
          dyn-events: [_ _ _ _ _] -> w97
          timeout: w100 -> [_ _ _ _ _]
          tunnel: w100 -> [_ _ _ w151 _]
          tunnel: [-1 -1 w149 w151 -1] -> w99
          tunnel: w98 -> [_ _ _ _ _]
          tunnel: [_ w123 w145 w157 w190] -> w94
          tunnel: [TRUE _ _ _ _] -> w93
          tunnel: [refnum<k21> refnum ("task out") w120 w148 w158 refnum<k21> refnum ("task out")] -> w92
          tunnel: [FALSE w118 w147 w156 FALSE] -> w91
          tunnel: w90 -> [_ _ w147 w154 _]
          tunnel: w89 -> [_ _ w148 w159 w191]
          tunnel: w88 -> [_ _ w149 w152 w187]
          tunnel: [FALSE w114 w146 w153 FALSE] -> w87
          tunnel: w86 -> [_ _ w146 w155 _]
          tunnel: [-1 w108 w149 w152 w187] -> w85
          event User Event {
            n169 = event-data() -> ()  [unwired: 1 in, 1 out]
          }
          event User Event {
            # "False: Ports\nTrue: Lines"
            n170 = event-data() -> ("DAQ Device Name"=w122:tag, "Digital Acquisition Parameters.Channels Ports Digital"=w121:tag[], "Digital Acquisition Parameters.Channels Lines Digital"=w119:tag[], "Digital Acquisition Parameters.Ports - Line"=w124:bool, "Digital Acquisition Parameters.Execution Task Frequency"=w110:u32)  [unwired: 1 in]
            n171 = call "Status Updated.vi"("Status"="Digital Acquisition Configured, ready in Helper Loop") -> ("error out"=w115:errorcluster)  [unwired: 10 in]
            n172 = case shown="False" w124 {
              tunnel: [w128 w138] -> w123
              tunnel: w122 -> [w134 w142]
              tunnel: w121 -> [w133 _]
              tunnel: [w131 w143] -> w120
              tunnel: w119 -> [_ w141]
              tunnel: [TRUE TRUE] -> w118
              tunnel: w115 -> [w126 w136]
              tunnel: [FALSE TRUE] -> w114
              frame False {
                n173 = call "Status Updated.vi"("Status"="Digital HL: Ports") -> ("error out"=w127:errorcluster)  [unwired: 10 in]
                n174 = call "DaqDigital_ConfigurationPorts.vi"("Canales"=w133, "DAQ Board Name"=w134) -> ("error out"=w132:errorcluster, "task out"=w131:refnum<k21>)  [unwired: 8 in]
                n175 = Merge Errors(w132, w127, w126) -> (w128:errorcluster)
              }
              frame True {
                n176 = call "Status Updated.vi"("Status"="Digital HL:Lines") -> ("error out"=w137:errorcluster)  [unwired: 10 in]
                n177 = call "DaqDigital_ConfigurationLines.vi"("Canales"=w141, "DAQ Board Name"=w142) -> ("error out"=w144:errorcluster, "task out"=w143:refnum<k21>)  [unwired: 8 in]
                n178 = Merge Errors(w144, w137, w136) -> (w138:errorcluster)
              }
            }
            n179 = Divide(x=1, y=w110) -> (x/y=w113:dbl)
            n180 = Multiply(x=w113, y=u32 1000) -> (x*y=w109:dbl)
            n181 = To Long Integer(number=w109) -> (32bit integer=w108:i32)
          }
          event User Event {
            n182 = event-data() -> ()  [unwired: 1 in, 1 out]
            n183 = call "Status Updated.vi"("Status"="Started Acquiring Digital Data") -> ("error out"=w145:errorcluster)  [unwired: 10 in]
          }
          event Timeout {
            n184 = event-data() -> ()  [unwired: 1 in, 1 out]
            n185 = case shown="True" w154 {
              tunnel: w159 -> [w162 w168]
              tunnel: [w162 w167] -> w158
              tunnel: [_ w166] -> w157
              tunnel: [w161 w163] -> w156
              tunnel: w154 -> [w161 w163]
              tunnel: w155 -> [w160 w165]
              tunnel: [w160 w164] -> w153
              frame False {
                # "This case determines whether the task has been configured, thus\nallows the system to start acquisition or ignores it."
              }
              frame True {
                n186 = case shown="True" w165 {
                  tunnel: w168 -> [w176 w183]
                  tunnel: [w175 w182] -> w167
                  tunnel: [w170 w178] -> w166
                  tunnel: w165 -> [w172 w180]
                  tunnel: [w172 w180] -> w164
                  frame False {
                    # "Ports"
                    n187 = call-poly <vilib>:"DAQmx Read.vi"("task/channels in"=w176) -> ("task out"=w175:refnum<k21>, "data"=w173:u32[], "error out"=w174:errorcluster)  [unwired: 12 in]
                    n188 = call "Converter_u32ToBoolArray.vi"("data"=w173) -> ("Boolean array"=w171:bool[])  [unwired: 10 in]
                    n189 = local write "Array Datos Digitales"(w171) -> ()
                    n190 = call "Digital Data Has Been Acquired.vi"("Digital Data Acq."=w171) -> ("error out"=w169:errorcluster)  [unwired: 10 in]
                    n191 = Merge Errors(w174, w169) -> (w170:errorcluster)
                  }
                  frame True {
                    # "Lines"
                    n192 = call-poly <vilib>:"DAQmx Read.vi"("task/channels in"=w183) -> ("task out"=w182:refnum<k21>, "data"=w179:bool[], "error out"=w181:errorcluster)  [unwired: 12 in]
                    n193 = local write "Array Datos Digitales"(w179) -> ()
                    n194 = call "Digital Data Has Been Acquired.vi"("Digital Data Acq."=w179) -> ("error out"=w177:errorcluster)  [unwired: 10 in]
                    n195 = Merge Errors(w181, w177) -> (w178:errorcluster)
                  }
                }
              }
            }
          }
          event User Event {
            n196 = event-data() -> ()  [unwired: 1 in, 1 out]
            n197 = call <vilib>:"DAQmx Clear Task.vi"("task in"=w191) -> ("error out"=w190:errorcluster)  [unwired: 14 in]
            n198 = call "Status Updated.vi"("Status"="Stopped Acquiring Digital Data") -> ()  [unwired: 10 in, 1 out]
          }
        }
        n199 = call-dynamic "Delacor_lib_QMH_Error Handler - Message Handling Loop.vi"("error in"=w94, "Message Queue in"=w95) -> ("dup error in"=w96:errorcluster)  [unwired: 8 in, 1 out]
      }
    }
    frame Error {
      # "Synchronize Caller Events.vi will inform Start Module.vi that the module has launched and will let the code calling Start Module.vi register for broadcasts and would permit the caller receive the broadcast that an error occurred at launch time."
      n200 = call-dynamic "Delacor_lib_QMH_Release Message Queue.vi"("error in"=w507, "Message Queue"=w505) -> ("error out"=w506:errorcluster)  [unwired: 9 in]
      n201 = call "Synchronize Caller Events.vi"("Singleton Module Admin in"=w508) -> ("error out"=w513:errorcluster)  [unwired: 9 in, 1 out]
      n202 = call "Module Name--constant.vi"() -> ("Module Name"=w511:string)  [unwired: 11 in]
      n203 = Format Into String(format string="An error occurred during initialization. %s is no longer running.", w511) -> (resulting string=w509:string)  [unwired: 2 in, 1 out]
      n204 = Merge Errors(w506, w513) -> (w514:errorcluster)
      n205 = call "Error Reported.vi"("Additional Information"=w509, "Error"=w514) -> ()  [unwired: 9 in, 1 out]
    }
  }
  n206 = Unregister For Events(event registration refnum=w12, error in=w11) -> (error out=w10:errorcluster)
  n207 = Unregister For Events(event registration refnum=w8, error in=w7) -> (error out=w6:errorcluster)
  n208 = Unregister For Events(event registration refnum=w5, error in=w4) -> (error out=w3:errorcluster)
  n209 = Merge Errors(w26, w29, w10, w6, w3) -> (w25:errorcluster)
  n210 = call "Close Module.vi"("error in (no error)"=w25, "Module Admin in"=w20) -> ("error out"=w27:errorcluster, "External Launch"=w14:bool, "Module Admin out"=w15:refnum<class "Delacor_lib_QMH_Module Admin.lvclass">)  [unwired: 7 in]
  n211 = Unregister For Events(event registration refnum=w19, error in=w27) -> (error out=w24:errorcluster)
  "error out" <- w24
  n212 = case "External Launch?" shown="True" w14 {
    tunnel: w24 -> [_ w515]
    frame False {
    }
    frame True {
      n213 = case shown="No Error" w515 {
        frame No Error {
          n214 = invoke class="VI" method="FP.Close"() -> ()  [unwired: 3 in, 3 out]
        }
        frame Error {
          n215 = invoke class="VI" method="FP.Open"("Activate"=TRUE ("Activate?")) -> ()  [unwired: 4 in, 5 out]
        }
      }
    }
  }
  n216 = local write "Module Admin"(w15) -> ()
